vi "add_NavSatStatus.vi"(3 "service":u16(ring)=1 items=["SERVICE_GPS"=1, "SERVICE_GLONASS"=2, "SERVICE_COMPASS"=4, "SERVICE_GALILEO"=8], 4 "status":i8(ring)=-1 items=["STATUS_NO_FIX"=-1, "STATUS_FIX"=0, "STATUS_SBAS_FIX"=1, "STATUS_GBAS_FIX"=2], 5 "msg in":string) -> (2 "msg out":string)   [LabVIEW 2014]
uses:
  std_msgs/subs/i8Scalar.vi
  std_msgs/subs/u16Scalar.vi
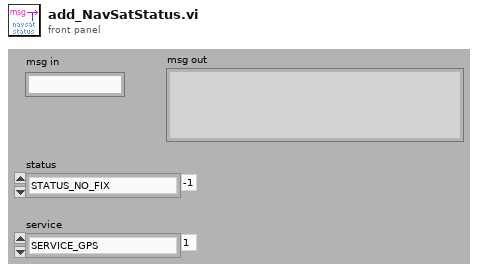
[diagram p1: front panel]
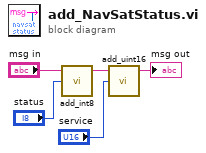
[diagram p0: block diagram]
diagram:
  n1 = call-poly "add_int8.vi"("Numeric"="status", "msg in"="msg in") -> ("msg out"=w4:string)  [unwired: 3 in]
  n2 = call-poly "add_uint16.vi"("Numeric"="service", "msg in"=w4) -> ("msg out"=→"msg out":string)  [unwired: 3 in]
